vi "Launcher Preparation.vi"(2 "Elevation":dbl, 3 "Shooting Motors":dbl) -> ()   [LabVIEW 2012]
uses:
  BotStatus.vi
  Motors Values.vi
  <vilib>/express/express arith-compare/Formula/XNode/ExpressFormulaBlockNode.xnode
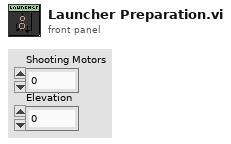
[diagram p1: front panel]
types:
  T1 = cluster{"Middle":bool, "InCannon":bool, "InFlipper":bool, "FlipperAtPlace":bool, "Bottom":bool, "FrisbeeDirection":bool}
  T2 = typedef "WPI_EncoderDevRef.ctl" = cluster{"DevStatus":errorcluster, "EncoderIndex":T3, "CounterIndex":T4, "DistancePerCount":dbl, "Decoding Type":T5}
  T3 = typedef "FPGA_EncoderIdx.ctl" = enum8{"Enc 0", "Enc 1", "Enc 2", "Enc 3", "Invalid"}
  T4 = typedef "FPGA_CounterCtrSystemIndex.ctl" = enum8{"Ctr 0", "Ctr 1", "Ctr 2", "Ctr 3", "Ctr 4", "Ctr 5", "Ctr 6", "Ctr 7", "Invalid"}
  T5 = typedef "WPI_EncoderType.ctl" = enum16{"1x", "2x", "4x"}
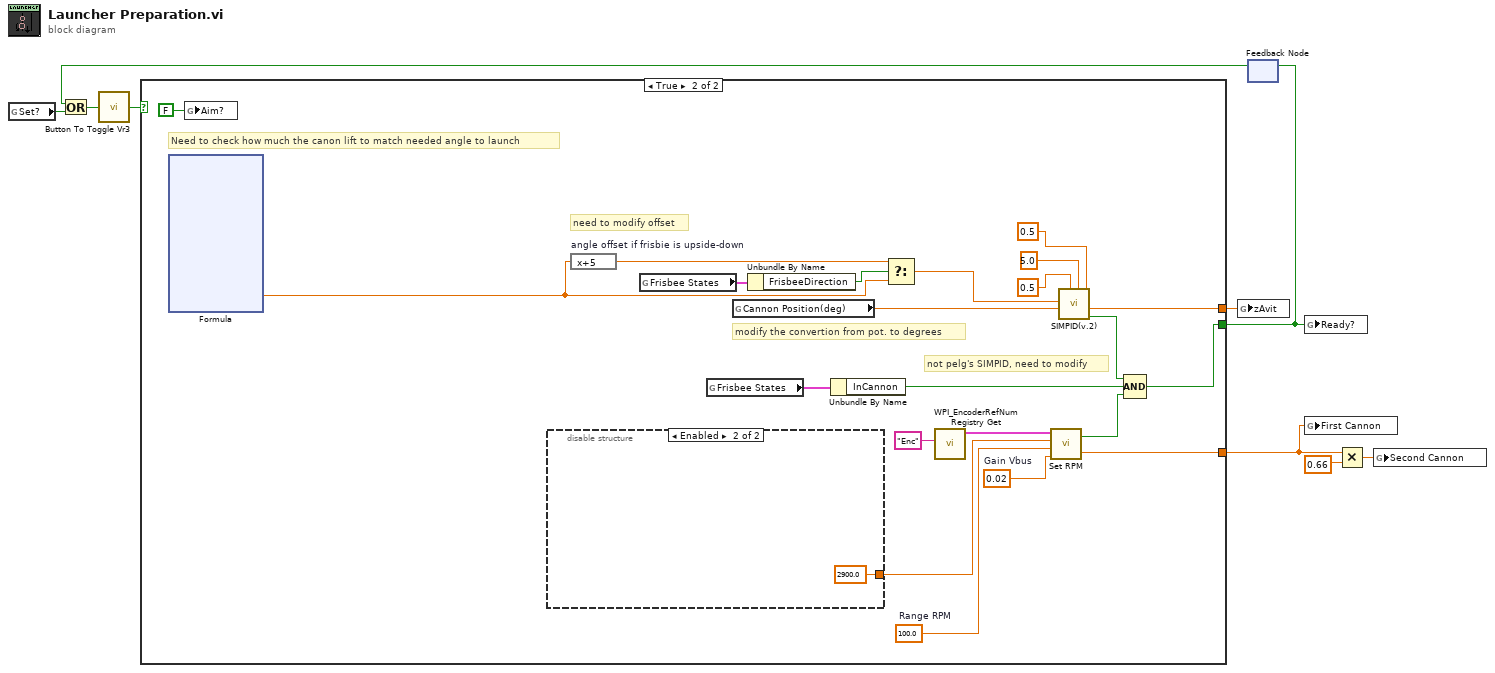
[diagram p0: block diagram]
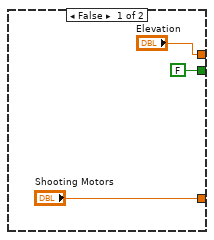
[diagram p2: hidden frame]
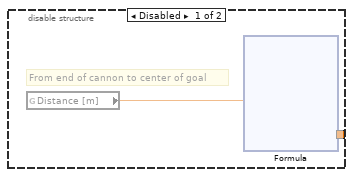
[diagram p3: hidden frame]
diagram:
  n1 = global read "BotStatus.vi" "Set?"() -> (w2:bool)
  n2 = feedback #1() -> (w1:bool)  [unwired: 1 in]
  n3 = Or(x=w1, y=w2) -> (x .or. y?=w5:bool)
  n4 = call "Button To Toggle Vr3.vi"("InValue"=w5) -> ("Result"=w4:bool)
  n5 = case shown="True" w4 {
    tunnel: ["Elevation" w25] -> w7
    tunnel: ["Shooting Motors" w23] -> w6
    tunnel: [FALSE w20] -> w3
    frame False {
    }
    frame True {
      w21 = 0.02  # Gain Vbus
      w22 = 100.0  # Range RPM
      # "need to modify offset"
      # "not pelg's SIMPID, need to modify"
      # "modify the convertion from pot. to degrees"
      # "Need to check how much the canon lift to match needed angle to launch"
      n6 = xnode "Formula"() -> ("Result"=w30:dbl)  [unwired: 5 in, 1 out]
      n7 = global write "BotStatus.vi" "Aim?"(FALSE ("Centerizing on Target")) -> ()
      n8 = disable-structure shown="Enabled" {
        disable-tunnel: [w35 2900.0 ("Set Point RPM")] -> w24
        frame Disabled {
          # "From end of cannon to center of goal"
          n9 = global read "BotStatus.vi" "Distance [m]"() -> (w36:dbl)
          n10 = xnode "Formula"("D"=w36) -> ("Result"=w35:dbl)  [unwired: 2 in, 1 out]
        }
        frame Enabled {
        }
      }
      n11 = expression code="x+5" "angle offset if frisbie is upside-down"(w30) -> (w29:dbl)
      n12 = global read "BotStatus.vi" "Frisbee States"() -> (w27:T1)
      n13 = global read "BotStatus.vi" "Frisbee States"() -> (w16:T1)
      n14 = global read "BotStatus.vi" "Cannon Position(deg)"() -> (w28:dbl)
      n15 = Unbundle By Name(w27) -> ("FrisbeeDirection"=w26:bool)
      n16 = Unbundle By Name(w16) -> ("InCannon"=w13:bool)
      n17 = Select(t=w29, s=w26, f=w30) -> (s? t:f=w31:dbl)
      n18 = call <vilib>:"WPI_EncoderRefNum Registry Get.vi"("refnum name"="Enc") -> ("EncoderDevRef"=w18:T2)  [unwired: 9 in, 1 out]
      n19 = call "Set RPM.vi"("Gain Vbus"=w21, "Range RPM"=w22, "Set Point RPM"=w24, "EncoderDevRef"=w18) -> ("Vbus Out"=w23:dbl, "READY!"=w14:bool)
      n20 = call "SIMPID(v.2).vi"("Range"=0.5, "upper limit"=5.0, "lower limit"=0.5, "Current Point"=w28, "Set Point"=w31) -> ("On Target"=w15:bool, "result"=w25:dbl)  [unwired: 5 in]
      n21 = Compound Arithmetic op=AND(w15, w13, w14) -> (w20:bool)
    }
  }
  n22 = global write "Motors Values.vi" "zAvit"(w7) -> ()
  n23 = feedback-in #1(w3) -> ()
  n24 = global write "BotStatus.vi" "Ready?"(w3) -> ()
  n25 = global write "Motors Values.vi" "First Cannon"(w6) -> ()
  n26 = Multiply(x=w6, y=0.66) -> (x*y=w8:dbl)
  n27 = global write "Motors Values.vi" "Second Cannon"(w8) -> ()
